vi "Display Logged Temp.vi"() -> ()   [LabVIEW 2015]
doc: "This VI is used as a subVI in the Temperature System exercise in the LabVIEW Basics I course."
uses:
  <vilib>/Utility/file.llb/Read From Spreadsheet File (DBL).vi
panel:
  in  "Return":bool
  out "Temperature Graph":T1(graph)
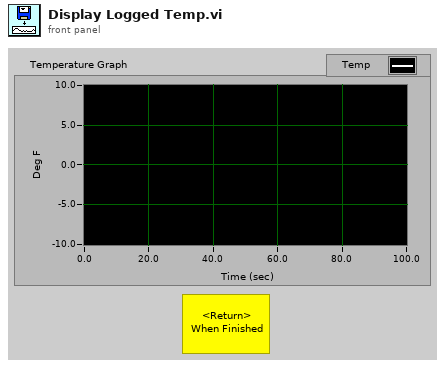
[diagram p1: front panel]
types:
  T1 = cluster{"Xo":i32, "Delta X":ext, "first row":dbl[]}
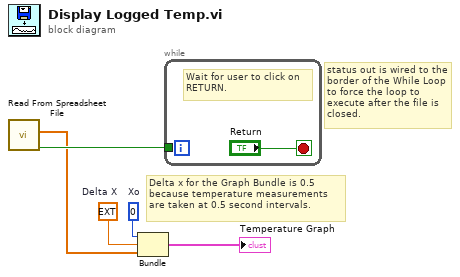
[diagram p0: block diagram]
diagram:
  w4 = ext 0.5  # Delta X
  w5 = 0  # Xo
  # "status out is wired to the border of the While Loop to force the loop to execute after the file is closed."
  # "Delta x for the Graph Bundle is 0.5\nbecause temperature measurements \nare taken at 0.5 second intervals."
  n1 = call-poly <vilib>:"Read From Spreadsheet File.vi"() -> ("EOF?"=w2:bool, "first row"=w1:dbl[])  [unwired: 7 in, 3 out]
  n2 = Bundle("Xo"=w5, "Delta X"=w4, "first row"=w1) -> (→"Temperature Graph":T1)  [unwired: 1 in]
  n3 = while {
    tunnel: w2 -> [_]
    stop <- "Return" stop-if-true
    # "Wait for user to click on\nRETURN."
  }
